vi "SimulatedDevice2.vi"() -> ()   [LabVIEW 2017]
uses:
  <vilib>/express/express analysis/Spectral/Block/exnSpectralBlock spectral measurements peak poly.vi
  <vilib>/express/express analysis/Spectral/Block/exnSpectralBlock spectral measurements peak DDT.vi
  <vilib>/express/express analysis/Spectral/XNode/ExpressSpectralMeasurementsBlockNode.xnode
panel:
  out "Subtraction FFT Graph":dynamicdata(graph)
  out "Addition FFT Graph":dynamicdata(graph)
  out "Subtraction Graph":dynamicdata(graph)
  out "Addition Graph":dynamicdata(graph)
  out "Signal #2":dynamicdata(graph)
  in  "Phase 2":dbl caption="Phase"
  in  "Offset 2":dbl caption="Offset"
  in  "Frequency 2":dbl=10.1 caption="Frequency"
  in  "Amplitude 2":dbl=1.0 caption="Amplitude"
  out "Signal #1":dynamicdata(graph)
  in  "Phase":dbl
  in  "Offset":dbl
  in  "Frequency":dbl=10.1
  in  "Amplitude":dbl=1.0
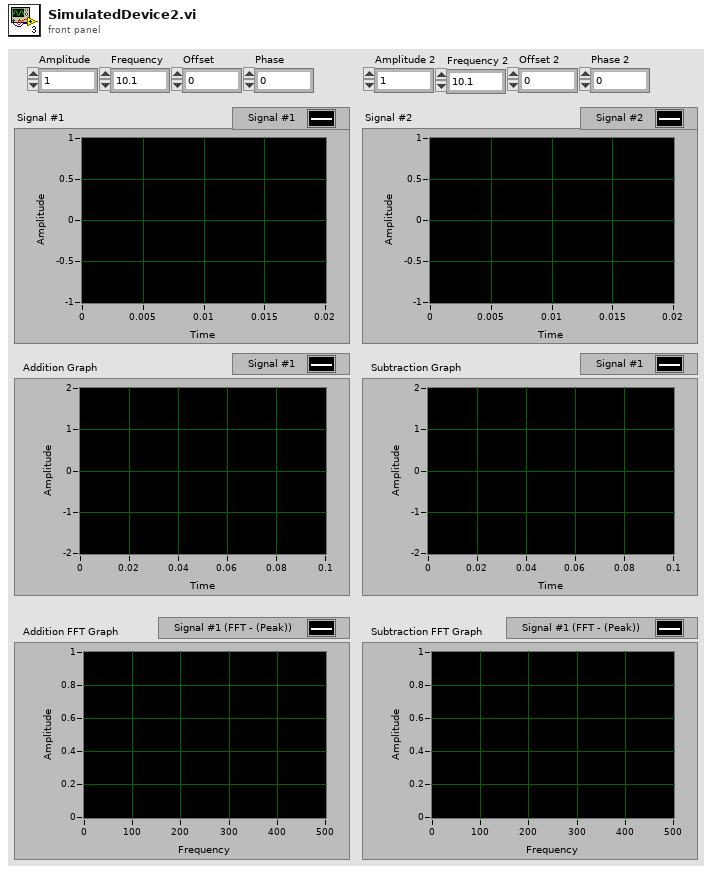
[diagram p1: front panel]
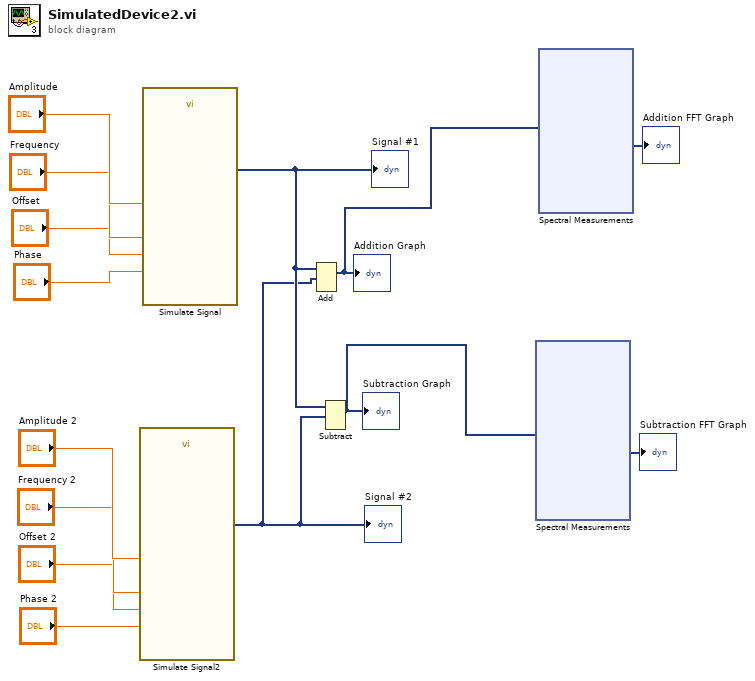
[diagram p0: block diagram]
diagram:
  n1 = call "Simulate Signal2"("Offset"="Offset 2", "Frequency"="Frequency 2", "Amplitude"="Amplitude 2", "Phase"="Phase 2") -> ("Signal #2"=w5:dynamicdata)  [unwired: 10 in, 1 out]
  "Signal #2" <- w5
  n2 = call "Simulate Signal"("Offset"="Offset", "Frequency"="Frequency", "Amplitude"="Amplitude", "Phase"="Phase") -> ("Signal #1"=w6:dynamicdata)  [unwired: 10 in, 1 out]
  "Signal #1" <- w6
  n3 = Add(1:w5, 2:w6) -> (0:w4:dynamicdata)  [unwired: 1 in, 1 out]
  "Addition Graph" <- w4
  n4 = Subtract(1:w5, 2:w6) -> (0:w2:dynamicdata)  [unwired: 1 in, 1 out]
  "Subtraction Graph" <- w2
  n5 = xnode "Spectral Measurements"("Signals"=w2) -> ("FFT - (Peak)"=→"Subtraction FFT Graph":dynamicdata)  [unwired: 1 in, 2 out]
  n6 = xnode "Spectral Measurements"("Signals"=w4) -> ("FFT - (Peak)"=→"Addition FFT Graph":dynamicdata)  [unwired: 1 in, 2 out]
